vi "HB_ImaqLLTriggeredGrab.vi"() -> ()   [LabVIEW 2009, in "HB_IMAQ_Examples.lvlib"]
doc: "The HL Grab VI acquires images continuously and displays the images in an image control using high-level acquisition VIs. A grab is appropriate for high-speed applications that process only one image at a time.\n\nIMAQ Init initializes the device. IMAQ Grab Setup initializes the grab function and starts capturing images to an internal software buffer. IMAQ Create creates an image buffer. IMAQ Grab Acquire copies the internal buffer to Image out, and an image control displays the image on the front panel. IMAQ Close releases resources associated with the acquisition, and IMAQ Dispose frees the image buffer."
uses:
  HB_IMAQ_Examples.lvlib
  <vilib>/vision/driver/IMAQdx.llb/IMAQdx Buffer Number Mode.ctl
  lib.lib/HGF_LVC/HGF_IMAQ/HGF_IMAQFactory/HGF_IMAQFactory.lvclass
  lib.lib/HGF_LVC/HGF_IMAQ/HGF_IMAQDevice/HGF_IMAQDevice.lvclass
  lib.lib/HGF_LVC/HGF_BaseClasses/HGF_Factory/HGF_Factory.lvclass
  lib.lib/HGF_LVC/HGF_DeviceBaseClasses/HGF_DeviceBase/HGF_DeviceBase.lvclass
  lib.lib/HGF_LVC/HGF_Auxiliary/HGF_Auxiliary.lvlib
  lib.lib/VisionTools/HGF_VisionTools/HGF_VisionTools.lvlib
  <vilib>/vision/driver/NI_Vision_Acquisition_Software.lvlib
panel:
  in  "Trigger Mode":T1(ring)=enum."Mode 0"
  out "Lost Counter":T2
  out "Last Valid Buffer Number":u32
  out "Last Valid Buffer Index":u32
  out "Acquiring?":bool
  in  "Skip trigger (linescan only)":u32
  in  "Delay":cluster{"Value":dbl, "Units":u32}={"Value"=0.0, "Units"=5} {"Units" items=["Scaled Encoder Counts"=4, "Milliseconds"=5]}
  in  "Activation":u32(ring) items=["Rising Edge", "Falling Edge", "AnyEdge", "LevelHigh", "LevelLow"]
  in  "Action":u32(ring) items=["Disabled", "Trigger start of acquisition", "Trigger start of each buffer list", "Trigger each buffer", "Trigger each line (linescan)", "Trigger end of acquisition"]
  in  "Frame timeout (ms)":u32=1000
  in  "Line Number":u32=2
  in  "Type":u32(ring) items=["External"=0, "RTSI"=1, "ISO In"=2, "Scaled Encoder"=5, "Software Trigger"=6]
  in  "Buffer Number Mode (Next)":T3
  out "error out":errorcluster
  in  "Number of buffers":u32=2
  out "processed FPS":dbl
  out "acquired FPS":dbl
  out "iteration":i32
  out "Image":T4(plugin-control)
  in  "interval / ms":u32=100
  in  "stop":bool
  in  "Image Type":T5 items=["Grayscale (U8)", "Grayscale (I16)", "Grayscale (SGL)", "Complex (CSG)", "RGB (U32)", "HSL (U32)", "RGB (U64)", "Grayscale (U16)"]
  in  "cameraName":string="HTCam_0"
  in  "imaqClassName":string="HGF_Prosilica_GC655"
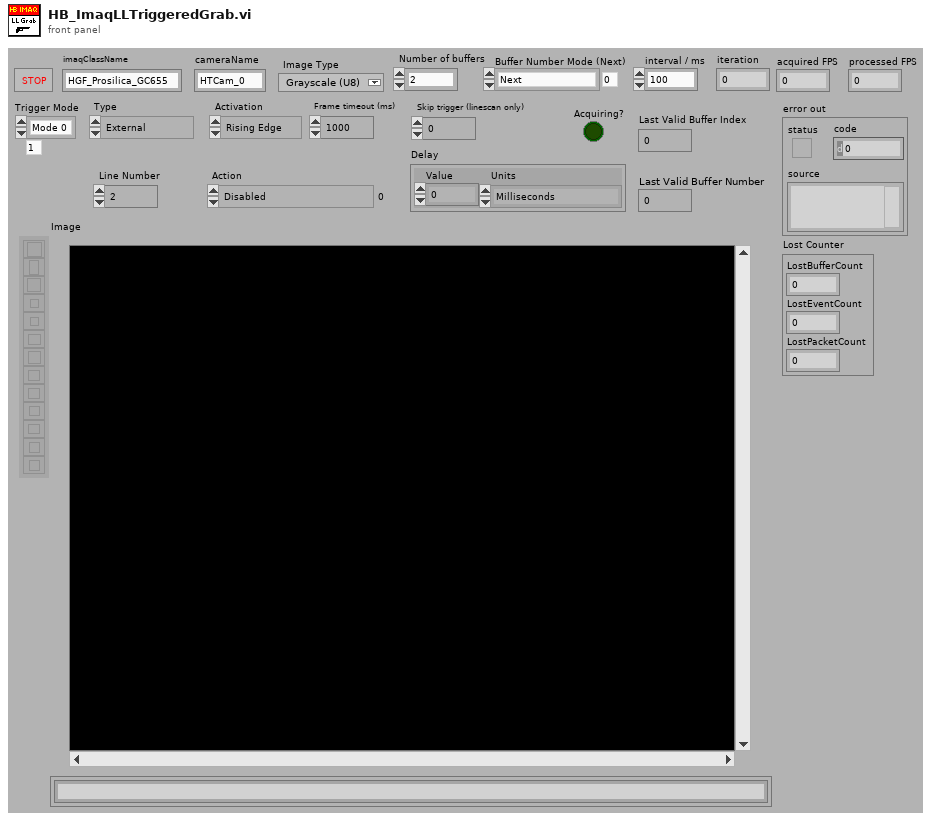
[diagram p1: front panel]
types:
  T1 = enum16{"Off", "Mode 0", "Mode 1", "Mode 2", "Mode 3", "Mode 4", "Mode 5"}
  T2 = cluster{"LostBufferCount":u32, "LostEventCount":u32, "LostPacketCount":u32}
  T3 = typedef "NI_Vision_Acquisition_Software.lvlib/IMAQdx Buffer Number Mode.ctl" = enum32{"Next", "Last", "Buffer Number"}
  T4 = typedef "IMAQ Image.ctl" = refnum<image>
  T5 = typedef "Image Type" = u32
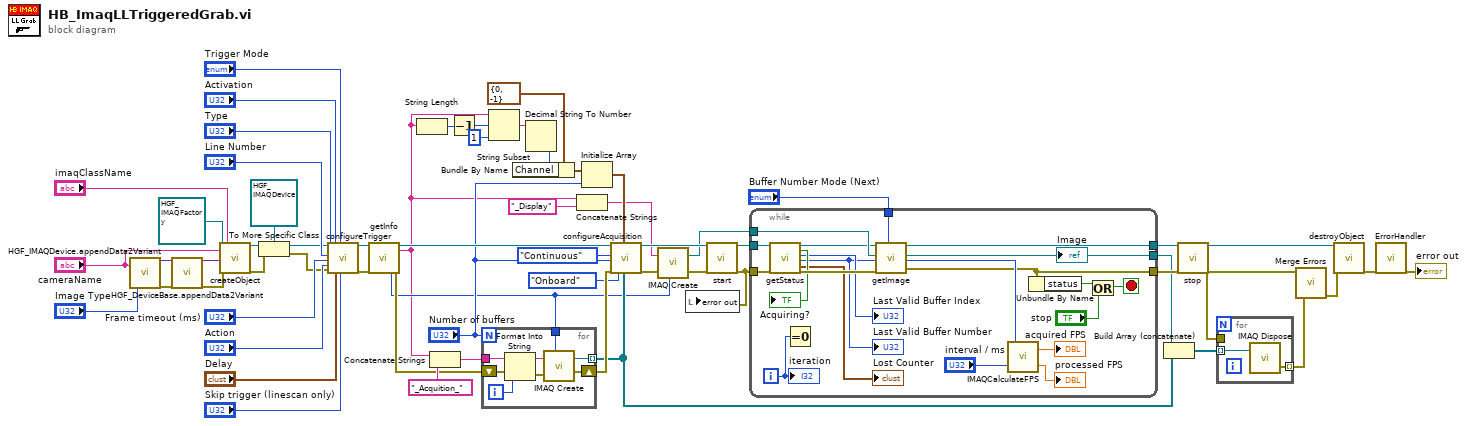
[diagram p0: block diagram]
diagram:
  n1 = call "HGF_IMAQDevice.appendData2Variant.vi"("cameraName"="cameraName", "imageType"="Image Type") -> ("dup initData"=w61:variant, "error out"=w60:errorcluster)  [unwired: 4 in, 12 out]
  n2 = call "HGF_DeviceBase.appendData2Variant.vi"("initData"=w61, "error in (no error)"=w60) -> ("dup initData"=w58:variant, "error out"=w59:errorcluster)  [unwired: 16 out]
  n3 = call "createObject.vi"("HGF_Factory"=refnum<class "HGF_IMAQFactory.lvclass"> refnum ("HGF_IMAQ.lvlib:HGF_IMAQFactory.lvclass"), "objectName"="cameraName", "initializationData"=w58, "error in (no error)"=w59, "className"="imaqClassName") -> ("HGF_Object"=w56:refnum<class "HGF_Factory.lvclass">, "error out"=w55:errorcluster)  [unwired: 13 out]
  n4 = To More Specific Class(target class=refnum<class "HGF_IMAQDevice.lvclass"> refnum ("HGF_IMAQ.lvlib:HGF_IMAQDevice.lvclass"), reference=w56, error in=w55) -> (specific class reference=w7:refnum<class "HGF_IMAQDevice.lvclass">, error out=w6:errorcluster)
  n5 = call "configureTrigger.vi"("HGF_IMAQDevice"=w7, "Type"="Type", "Line Number (0)"="Line Number", "Frame timeout (ms)"="Frame timeout (ms)", "Action"="Action", "error in (no error)"=w6, "Activation"="Activation", "Delay (0ms)"="Delay", "Mode (off)"="Trigger Mode", "Skip trigger (linescan only) (0)"="Skip trigger (linescan only)") -> ("dup HGF_IMAQDevice"=w17:refnum<class "HGF_IMAQDevice.lvclass">, "error out"=w16:errorcluster)  [unwired: 8 in]
  n6 = call "getInfo.vi"("HGF_IMAQDevice"=w17, "error in (no error)"=w16) -> ("imageType"=w3:T5, "dup HGF_IMAQDevice"=w45:refnum<class "HGF_IMAQDevice.lvclass">, "cameraName"=w2:string, "error out"=w43:errorcluster)  [unwired: 12 in, 2 out]
  n7 = String Length(string=w2) -> (length=w28:i32)
  n8 = Concatenate Strings(w2, "_Acquition_" ("string")) -> (w44:string)
  n9 = Decrement(x=w28) -> (x-1=w27:i32)
  n10 = for {
    N: "Number of buffers" -> [_]
    tunnel: w3 -> [w69]
    tunnel: w44 -> [w67]
    shift-right: [w68] -> w49
    shift-left: w43 -> [w65]
    tunnel: [w62] -> w38 mode=indexing
    i -> [w63]
    n11 = Format Into String(initial string=w67, error in=w65, w63) -> (resulting string=w66:string, error out=w64:errorcluster)  [unwired: 1 in]
    n12 = call "IMAQ Create"("Image Name"=w66, "Image Type"=w69, "error in (no error)"=w64) -> ("New Image"=w62:T4, "error out"=w68:errorcluster)  [unwired: 1 in, 1 out]
  }
  n13 = String Subset(string=w2, offset (0)=w27, length (rest)=1 ("length (rest)")) -> (substring=w24:string)
  n14 = Decimal String To Number(string=w24) -> (number=w23:i32)  [unwired: 3 out]
  n15 = Bundle By Name(cluster=cluster{"Skip Count":u32, "Channel":i32} {"Skip Count"=0, "Channel"=-1} ("Buffer Parameter"), "Channel"=w23) -> (w22:cluster{"Skip Count":u32, "Channel":i32})
  n16 = Concatenate Strings(w2, "_Display" ("string")) -> (w4:string)
  n17 = Initialize Array(w22, "Number of buffers") -> (w20:cluster{"Skip Count":u32, "Channel":i32}[])
  n18 = call "configureAcquisition.vi"("HGF_IMAQDevice"=w45, "Continuous?"=enum16{"One-Shot", "Continuous"}."Continuous", "Number of buffers"="Number of buffers", "error in (no error)"=w49, "Memory Location"=enum16{"System", "Onboard"}."Onboard", "Buffer Parameters"=w20, "Image Array"=w38) -> ("dup HGF_IMAQDevice"=w42:refnum<class "HGF_IMAQDevice.lvclass">, "error out"=w1:errorcluster)  [unwired: 11 in]
  n19 = call "IMAQ Create"("Image Name"=w4, "Image Type"=w3, "error in (no error)"=w1) -> ("New Image"=w39:T4, "error out"=w40:errorcluster)  [unwired: 1 in, 1 out]
  n20 = call "start.vi"("HGF_IMAQDevice"=w42, "error in (no error)"=w40) -> ("dup HGF_IMAQDevice"=w41:refnum<class "HGF_IMAQDevice.lvclass">, "error out"=w9:errorcluster)  [unwired: 16 in]
  n21 = local write "error out"(w9) -> ()
  n22 = while {
    tunnel: w41 -> [w84]
    tunnel: w9 -> [w82]
    tunnel: w39 -> [w86]
    tunnel: [w70] -> w34
    tunnel: [w71] -> w35
    tunnel: [w87] -> w37
    tunnel: "Buffer Number Mode (Next)" -> [w85]
    i -> [w72]
    stop <- w88 stop-if-true
    n23 = call "getStatus.vi"("HGF_IMAQDevice"=w84, "error in (no error)"=w82) -> ("Lost Counter"=→"Lost Counter":T2, "dup HGF_IMAQDevice"=w83:refnum<class "HGF_IMAQDevice.lvclass">, "Acquiring?"=→"Acquiring?":bool, "Last Valid Buffer Index"=→"Last Valid Buffer Index":u32, "Last Valid Buffer Number"=w73:u32, "error out"=w81:errorcluster)  [unwired: 12 in]
    "Last Valid Buffer Number" <- w73
    n24 = Equal To 0?(x=w72) -> ()  [unwired: 1 out]
    n25 = call "getImage.vi"("HGF_IMAQDevice"=w83, "Image In"=w86, "Buffer Number"=w73, "error in (no error)"=w81, "Buffer Number Mode (Next)"=w85) -> ("dup HGF_IMAQDevice"=w87:refnum<class "HGF_IMAQDevice.lvclass">, "Image Out"=w70:T4, "Buffer Number Copied"=w77:i32, "error out"=w71:errorcluster)  [unwired: 8 in, 3 out]
    "Image" <- w70
    n26 = call "IMAQCalculateFPS.vi"("Update interval"="interval / ms", "buffer number"=w77) -> ("processed FPS"=→"processed FPS":dbl, "acquired FPS"=→"acquired FPS":dbl)
    n27 = Unbundle By Name(w71) -> ("status"=w90:bool)
    n28 = Or(x=w90, y="stop") -> (x .or. y?=w88:bool)
    "iteration" <- w72
  }
  n29 = Build Array (concatenate)(w34, w38) -> (w33:T4[])
  n30 = call "stop.vi"("HGF_IMAQDevice"=w37, "error in (no error)"=w35) -> ("dup HGF_IMAQDevice"=w36:refnum<class "HGF_IMAQDevice.lvclass">, "error out"=w32:errorcluster)  [unwired: 16 in]
  n31 = for {
    tunnel: [w92] -> w31 mode=indexing
    tunnel: w32 -> [_]
    tunnel: w33 -> [w91] mode=indexing
    n32 = call "IMAQ Dispose"("Image"=w91) -> ("error out"=w92:errorcluster)  [unwired: 2 in, 3 out]
  }
  n33 = call <vilib>:"Merge Errors.vi"("error array in"=w31, "error in 1 (no error)"=w32) -> ("error out"=w30:errorcluster)  [unwired: 2 in, 3 out]
  n34 = call "destroyObject.vi"("HGF_Factory"=w36, "error in (no error)"=w30) -> ("error out"=w53:errorcluster)  [unwired: 17 out]
  n35 = call "ErrorHandler.vi"("error in (no error)"=w53) -> ("error out"=→"error out":errorcluster)  [unwired: 6 in, 12 out]
